vi "SPCResetTrigger.vi"(1 "error in (no error)":errorcluster) -> (0 "error out":errorcluster)   [LabVIEW 2009]
uses:
  AO Update Channel (scaled value).vi
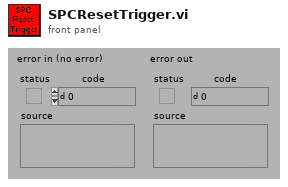
[diagram p1: front panel]
types:
  T1 = typedef "AnalogSettings.ctt" = cluster{"PCI 671x Device Number":u32, "Samples per Unit":u32}
  T2 = typedef "SPCConfiguration.ctt" = cluster{"SPC Initialization File":path, "Module Number":u16, "Operation Mode":u16, "Trigger Channel":tag}
  T3 = typedef "FIFOSettings.ctt" = cluster{"Measurement":cluster{"Binning (ms)":sgl, "External Trigger Condition":u16, "Stop Condition:":u16, "Stop Count":dbl, "Buffer Size (Photons)":u32, "No of Channels":u16, "Ext Latch Delay":i16}, "ADC":cluster{"Binning (HH)":i16, "Dither Range":i16, "Count Increment":i16, "Mode":u16}, "SYNC":cluster{"SYNC ZC Level (mV)":sgl, "SYNC Freq Divider":u16, "SYNC Holdoff (ps)":sgl, "SYNC Threshold (mV)":sgl}, "TAC":cluster{"TAC Range (ns)":sgl, "TAC Gain":i16, "TAC Offset (%)":sgl, "TAC Limit Low (%)":sgl, "TAC Limit High (%)":sgl}, "Ch 2":cluster{"Ch2 ZC Level (mV)":sgl, "Ch2 Holdoff (ps)":sgl, "Ch2 Threshold (mV)":sgl}, "Ch 3":cluster{"Ch3 ZC Level (mV)":sgl, "Ch3 Holdoff (ps)":sgl, "Ch3 Threshold (mV)":sgl}, "Ch 4":cluster{"Ch4 ZC Level (mV)":sgl, "Ch4 Holdoff (ps)":sgl, "Ch4 Threshold (mV)":sgl}, "Ch1":cluster{"Ch1 ZC Level (mV)":sgl, "Ch1 Holdoff (ps)":sgl, "Ch1 Threshold (mV)":sgl}}
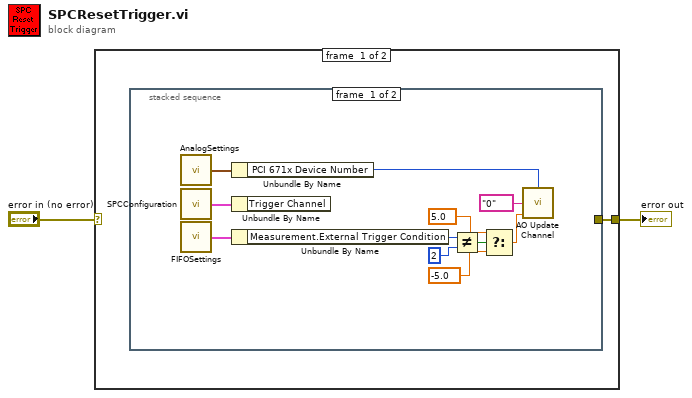
[diagram p0: block diagram]
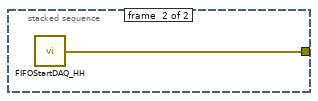
[diagram p2: hidden frame]
diagram:
  n1 = case shown="No Error" "error in (no error)" {
    selector: "error in (no error)" -> [_ w16]
    tunnel: [w3 w16] -> w1
    frame #0 {
      n2 = stacked-sequence {
        tunnel: [_ w15] -> w3
        frame #0 {
          n3 = call "AnalogSettings.vi"() -> ("Analog Settings (output)"=w13:T1)  [unwired: 2 in]
          n4 = call "SPCConfiguration.vi"() -> ("SPC Configuration (output)"=w14:T2)  [unwired: 2 in]
          n5 = call "FIFOSettings.vi"() -> ("FIFO Settings(out)"=w12:T3)  [unwired: 2 in]
          n6 = Unbundle By Name(w13) -> ("PCI 671x Device Number"=w6:u32)
          n7 = Unbundle By Name(w14) -> ()  [unwired: 1 out]
          n8 = Unbundle By Name(w12) -> ("Measurement.External Trigger Condition"=w11:u16)
          n9 = Not Equal?(x=w11, y=u16 2) -> (x != y?=w5:bool)
          n10 = Select(t=5.0, s=w5, f=-5.0) -> (s? t:f=w7:dbl)
          n11 = call-poly "AO Update Channel.vi"("value"=w7, "channel (0)"=tag "0", "device"=w6) -> ()
        }
        frame #1 {
          n12 = call "FIFOStartDAQ_HH.vi"() -> ("error out"=w15:errorcluster)  [unwired: 1 in]
        }
      }
    }
    frame #1 {
    }
  }
  "error out" <- w1
